vi "Read SubPnl for Display.vi"(8 "error in (no error)":errorcluster, 11 "HIJ Vision Application in":refnum<class "HIJ Vision Application.lvclass">) -> (0 "error out":errorcluster, 2 "SubPnl for Display":refnum<vi>, 3 "HIJ Vision Application out":refnum<class "HIJ Vision Application.lvclass">)   [LabVIEW 2014, in "HIJ Vision Application.lvlib" / "HIJ Vision Application.lvclass"]
uses:
  HIJ Vision Application.lvclass
  HIJ Vision Application.lvclass/HIJ Vision Application.ctl
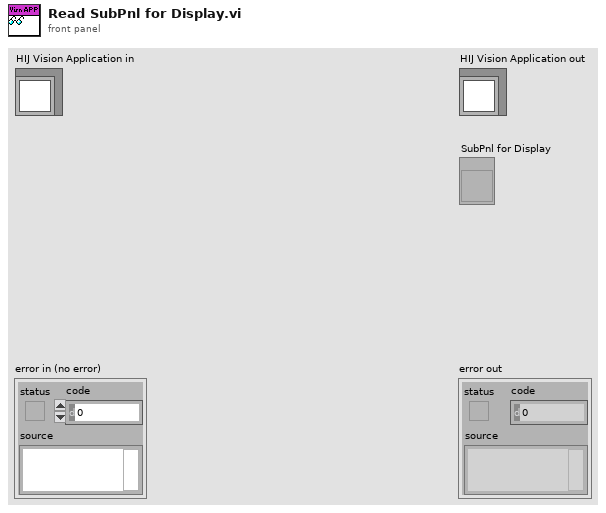
[diagram p1: front panel]
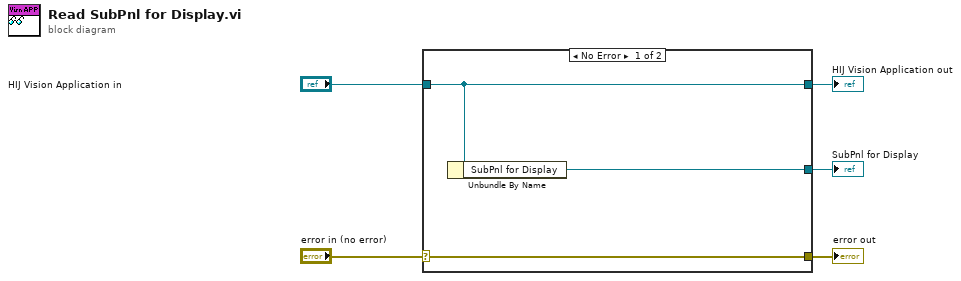
[diagram p0: block diagram]
diagram:
  n1 = case shown="No Error" "error in (no error)" {
    selector: "error in (no error)" -> [w8 w9]
    tunnel: [w8 w9] -> w4
    tunnel: [w7 w10] -> w2
    tunnel: "HIJ Vision Application in" -> [w7 w10]
    tunnel: [w6 _] -> w1
    frame No Error {
      n2 = Unbundle By Name(w7) -> ("SubPnl for Display"=w6:refnum<vi>)
    }
    frame Error {
    }
  }
  "error out" <- w4
  "HIJ Vision Application out" <- w2
  "SubPnl for Display" <- w1
